vi "Create 2dStringArrayMsg.vi"(8 "error in (no error)":errorcluster, 10 "Message Data":string[][](array[string]), 11 "Message Name":string) -> (0 "error out":errorcluster, 3 "2dStringArrayMsg Out":refnum<class "2dStringArrayMsg.lvclass">)   [LabVIEW 2018, in "LapDog.Messaging.v3.NativeArrays.lvlib" / "2dStringArrayMsg.lvclass"]
doc: "Returns a 2dStringArrayMsg object with the given name.\n\nThis method executes regardless of the error in state."
uses:
  2dStringArrayMsg.lvclass
  T:/git/LapDog.Messaging/src/LapDog.Messaging/Message/Message.lvclass
  2dStringArrayMsg.lvclass/2dStringArrayMsg.ctl
  LapDog.Messaging/Message/Message.lvclass
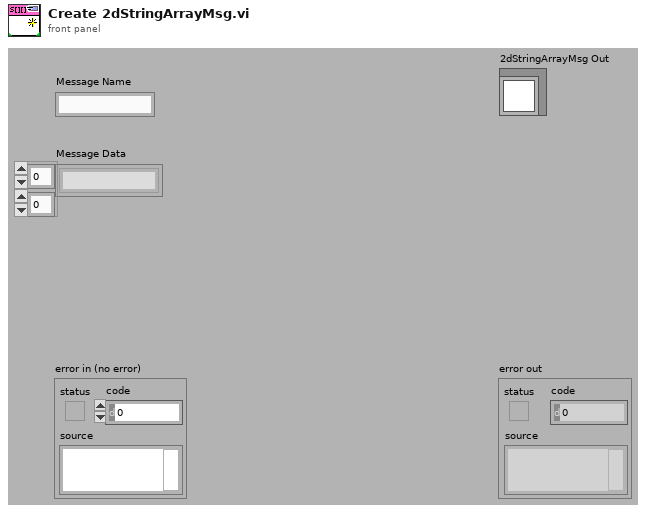
[diagram p1: front panel]
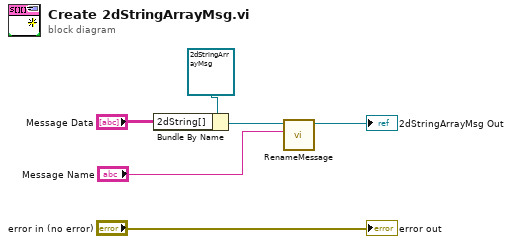
[diagram p0: block diagram]
diagram:
  n1 = Bundle By Name(cluster=refnum<class "2dStringArrayMsg.lvclass"> refnum ("StringMsg in"), "2dString[]"="Message Data") -> (w4:refnum<class "2dStringArrayMsg.lvclass">)
  n2 = call "RenameMessage.vi"("Message Name"="Message Name", "Message in"=w4) -> ("Message out"=→"2dStringArrayMsg Out":refnum<class "2dStringArrayMsg.lvclass">)  [unwired: 8 in, 1 out]
  "error out" <- "error in (no error)"
